vi "niDDC Send Software Trigger.vi"(8 "error in (no error)":errorcluster, 11 "Class in":refnum<class "7976R_v1.lvclass">) -> (0 "error out":errorcluster, 3 "Class out":refnum<class "7976R_v1.lvclass">)   [LabVIEW 2015, in "7976R_v1.lvclass"]
uses:
  <userlib>/SE-APP-Receiver/NI5772/7976R_v1/7976R_v1.lvclass
  <userlib>/SE-APP-Receiver/NI5772/7976R_v1/Private/FPGA VI Reference_DDC_v1.8.ctl
  <vilib>/rvi/interface/nirviReadWriteControl/nirviReadWriteControl.xnode
  NiFpgaLv.dll
  <vilib>/Utility/error.llb/Error Cluster From Error Code.vi
  <vilib>/rvi/interface/Simulation/niFpgaSimulationCallBeginRW.vi
  <vilib>/rvi/errors/niLvFpgaAdjustHostInterfaceError.vi
panel:
  in  "seconds to read":dbl=0.001 format="%#_13p"
  in  "trig.sw start trigger":bool
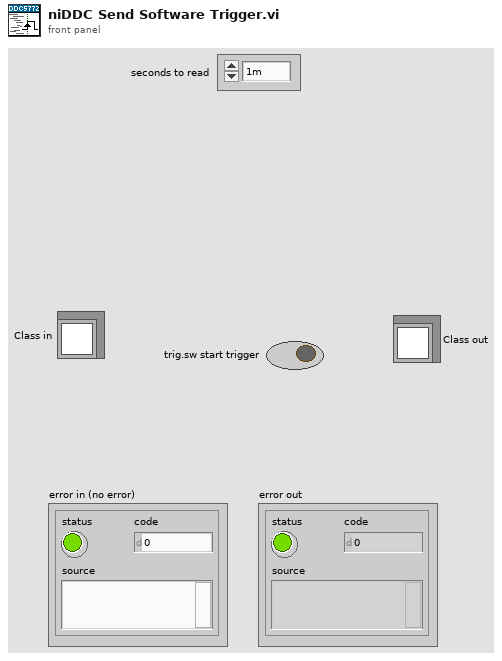
[diagram p1: front panel]
types:
  T1 = typedef "7976R_v1.lvclass/FPGA VI Reference_DDC_v1.8.ctl" = refnum<k20>
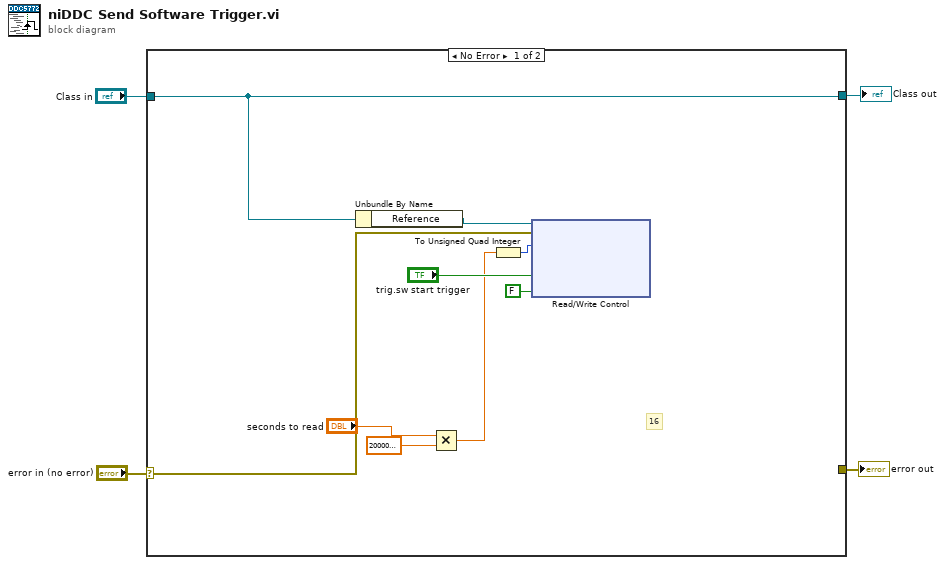
[diagram p0: block diagram]
diagram:
  n1 = case shown="No Error" "error in (no error)" {
    selector: "error in (no error)" -> [w5 w15]
    tunnel: [_ w15] -> w4
    tunnel: "Class in" -> [w6 w14]
    tunnel: [w6 w14] -> w1
    frame No Error {
      w13 = FALSE
      # "16"
      n2 = Unbundle By Name(w6) -> ("Reference"=w8:T1)
      n3 = Multiply(x="seconds to read", y=200000000.0) -> (x*y=w9:dbl)
      n4 = To Unsigned Quad Integer(1:w9) -> (0:w10:u64)
      n5 = xnode "Read/Write Control"("FPGA VI Reference In"=w8, "error in"=w5, "trig.samples.to.acq"=w10, "trig.sw start trigger"=w13, "trig.sw start trigger"="trig.sw start trigger", "trig.sw start trigger"=w13) -> ()  [unwired: 2 out]
    }
    frame Error {
    }
  }
  "error out" <- w4
  "Class out" <- w1
